vi "AggregationRate.vi"   [LabVIEW 2018, in "OXYGEN.lvlib"]
uses:
  OXYGEN.lvlib
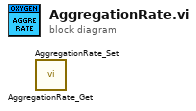
[diagram p0: block diagram]
diagram:
  n1 = call "AggregationRate_Get.vi"() -> ()  [unwired: 8 in, 4 out]
  n2 = call "AggregationRate_Set.vi"() -> ()  [unwired: 9 in, 3 out]
